vi "Prompt for Replacement.vi"(6 "Calling VI in":refnum<vi>, 8 "error in (no error)":errorcluster) -> (0 "error out":errorcluster, 2 "OK?":bool, 3 "Replace Info":T1={"Filter Column"=enum."Description", "Filter Type"=enum."Contains", "Filter Value"="", "Case Sensitive?"=FALSE, "Replace Column"=enum."Description", "Replace Value"=""})   [LabVIEW 2020, in "VI Properties Editor.lvlib"]
doc: "Displays a window to find and replace item properties."
uses:
  VI Properties Editor.lvlib
  CTLs/Filter Column.ctl
  CTLs/Filter Type.ctl
  CTLs/Replace Column.ctl
  CTLs/Replace Info.ctl
panel:
  in  "Case Sensitive?":bool caption="Case sensitive"
  in  "Replace Column Enum":T4
  in  "Replace Column":u16(ring) caption="Replacement Column" items=["Window Title", "Description", "Help Path", "Help Tag", "Custom Title?", "Help URL", "Help Type", "Control Label", "Control Caption", "Control Description", "Control Tip Strip"]
  in  "Replacement Value":string
  in  "Cancel":bool
  in  "OK":bool
  in  "Filter Type Enum":T3
  in  "Filter Type":u16(ring) items=["Contains", "Equals", "Starts with", "Ends with", "Is empty", "Does not contain", "Does not equal", "Is not empty"]
  in  "Filter Column":u16(ring) items=["Name", "Path", "Type", "Window Title", "Description", "Help Path", "Help Tag", "Custom Title?", "Reentrancy", "Inlined?", "Help URL", "Help Type", "Allow Debugging?", "Auto Error Handling?", "Run When Opened?", "Suspend When Called?", "Priority", "Preferred Exec Sytem", "Control Label", "Control Caption", "Control Description", "Control Tip Strip"]
  in  "Filter Value":string
  in  "Filter Column Enum":T2
  # "Find VIs or controls where"
  # "and change the following property to the following value:"
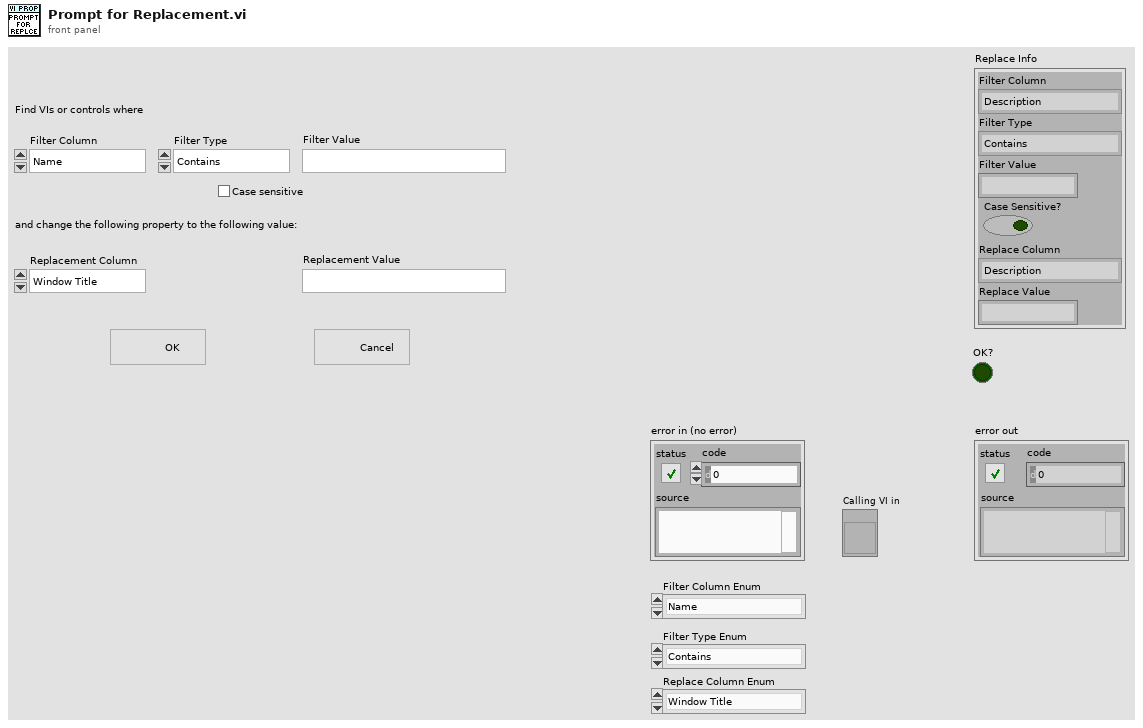
[diagram p1: front panel]
types:
  T1 = typedef "VI Properties Editor.lvlib/Replace Info.ctl" = cluster{"Filter Column":T2, "Filter Type":T3, "Filter Value":string, "Case Sensitive?":bool, "Replace Column":T4, "Replace Value":string}
  T2 = typedef "VI Properties Editor.lvlib/Filter Column.ctl" = enum16{"Name", "Path", "Type", "Window Title", "Description", "Help Path", "Help Tag", "Custom Title?", "Reentrancy", "Inlined?", "Help URL", "Help Type", "Allow Debugging?", "Auto Error Handling?", "Run When Opened?", "Suspend When Called?", "Priority", "Preferred Exec Sytem", "Control Label", "Control Caption", "Control Description", "Control Tip Strip"}
  T3 = typedef "VI Properties Editor.lvlib/Filter Type.ctl" = enum16{"Contains", "Equals", "Starts with", "Ends with", "Is empty", "Does not contain", "Does not equal", "Is not empty"}
  T4 = typedef "VI Properties Editor.lvlib/Replace Column.ctl" = enum16{"Window Title", "Description", "Help Path", "Help Tag", "Custom Title?", "Help URL", "Help Type", "Control Label", "Control Caption", "Control Description", "Control Tip Strip"}
  T5 = enum32{"Invalid", "Standard", "Closed", "Hidden", "Minimized", "Maximized"}
  T6 = enum8{"Enabled", "Disabled", "Disabled and Grayed Out"}
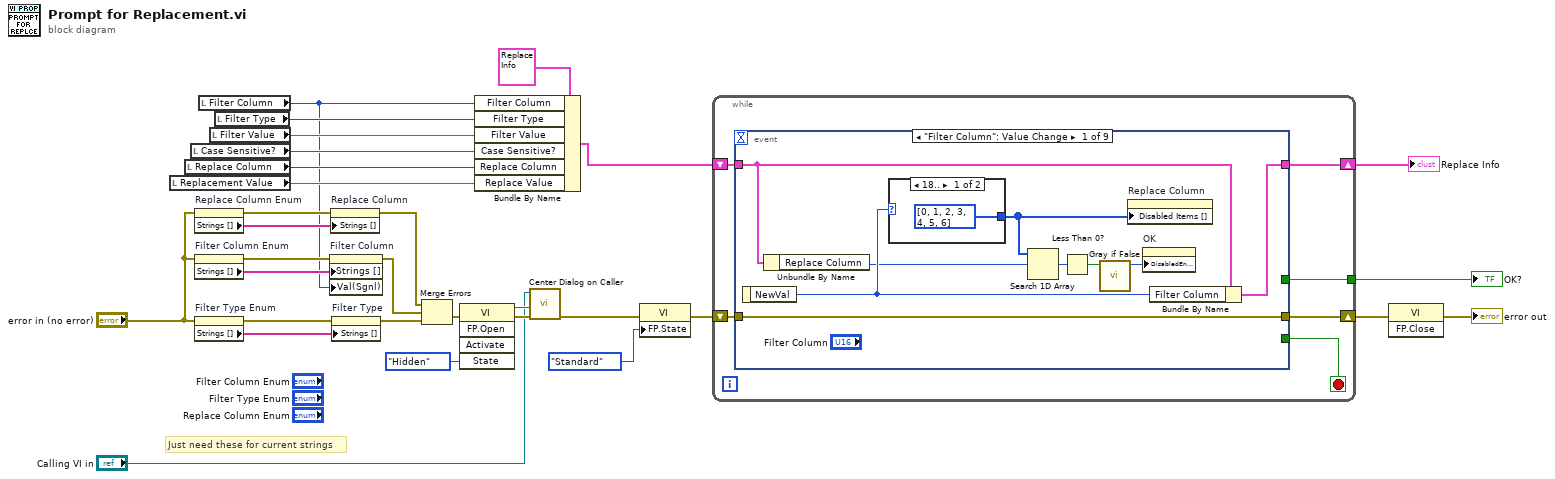
[diagram p0: block diagram]
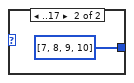
[diagram p2: hidden frame]
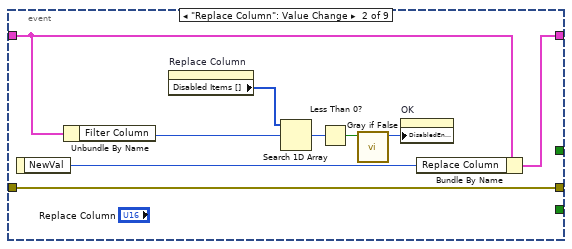
[diagram p3: hidden frame]
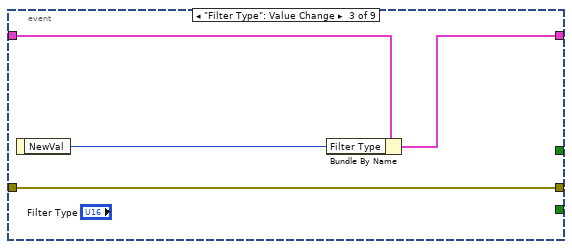
[diagram p4: hidden frame]
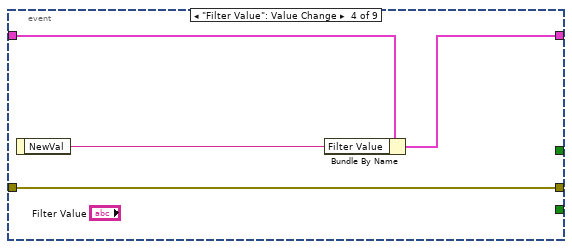
[diagram p5: hidden frame]
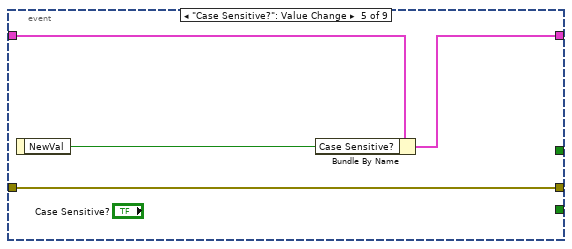
[diagram p6: hidden frame]
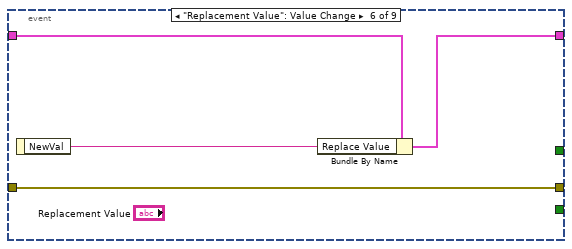
[diagram p7: hidden frame]
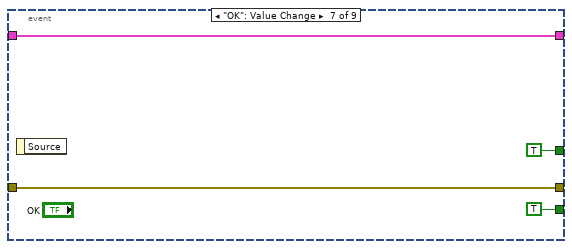
[diagram p8: hidden frame]
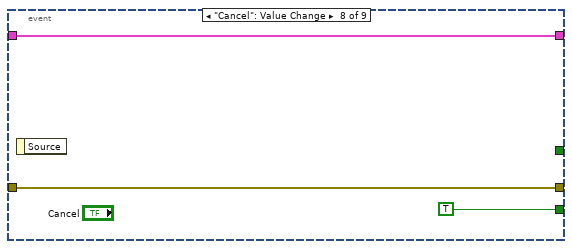
[diagram p9: hidden frame]
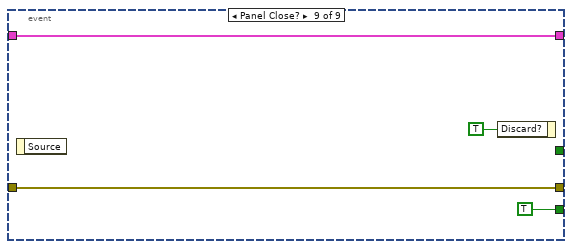
[diagram p10: hidden frame]
diagram:
  # "Just need these for current strings"
  n1 = local read "Replacement Value"() -> (w6:string)
  n2 = local read "Replace Column"() -> (w7:u16)
  n3 = local read "Case Sensitive?"() -> (w2:bool)
  n4 = property on="Replace Column Enum" class="Enum (strict)"(error in="error in (no error)") -> (error out=w18:errorcluster, "Strings []"=w5:string[])  [unwired: 1 in, 1 out]
  n5 = property on="Filter Column Enum" class="Enum (strict)"(error in="error in (no error)") -> (error out=w30:errorcluster, "Strings []"=w9:string[])  [unwired: 1 in, 1 out]
  n6 = property on="Filter Type Enum" class="Enum (strict)"(error in="error in (no error)") -> (error out=w29:errorcluster, "Strings []"=w17:string[])  [unwired: 1 in, 1 out]
  n7 = local read "Filter Column"() -> (w1:u16)
  n8 = local read "Filter Value"() -> (w15:string)
  n9 = local read "Filter Type"() -> (w14:u16)
  n10 = property on="Filter Column" class="Ring (strict)"(error in=w30, "Strings []"=w9, "Val(Sgnl)"=w1) -> (error out=w28:errorcluster)  [unwired: 1 in, 1 out]
  n11 = property on="Replace Column" class="Ring (strict)"(error in=w18, "Strings []"=w5) -> (error out=w19:errorcluster)  [unwired: 1 in, 1 out]
  n12 = property on="Filter Type" class="Ring (strict)"(error in=w29, "Strings []"=w17) -> (error out=w27:errorcluster)  [unwired: 1 in, 1 out]
  n13 = Merge Errors(w19, w28, w27) -> (w22:errorcluster)
  n14 = invoke on="Invoke Node" class="VI" method="FP.Open"(error in=w22, "State"=T5."Hidden") -> (reference out=w12:refnum<vi>, error out=w23:errorcluster)  [unwired: 3 in, 3 out]
  n15 = Bundle By Name(cluster=T1 {"Filter Column"=enum."Description", "Filter Type"=enum."Contains", "Filter Value"="", "Case Sensitive?"=FALSE, "Replace Column"=enum."Description", "Replace Value"=""} ("Replace Info"), "Filter Column"=w1, "Filter Type"=w14, "Filter Value"=w15, "Case Sensitive?"=w2, "Replace Column"=w7, "Replace Value"=w6) -> (w4:T1)
  n16 = call "Center Dialog on Caller.vi"("error in (no error)"=w23, "Dialog VI"=w12, "Calling VI in"="Calling VI in") -> ("error out"=w24:errorcluster)  [unwired: 7 in, 1 out]
  n17 = property on="Property Node" class="VI"(error in=w24, "FP.State"=T5."Standard" ("Front Panel Window:State")) -> (error out=w21:errorcluster)  [unwired: 1 in, 1 out]
  n18 = while {
    tunnel: [w31] -> w16
    shift-right: [w33] -> w3
    shift-left: w4 -> [w34]
    shift-right: [w35] -> w26
    shift-left: w21 -> [w36]
    stop <- w32 stop-if-true
    n19 = event shown="[0] \"Filter Column\": Value Change" {
      selector: _ -> [_ _ _ _ _ _ _ _ _]
      dyn-events: _ -> [_ _ _ _ _ _ _ _ _]
      timeout: _ -> [_ _ _ _ _ _ _ _ _]
      tunnel: w34 -> [w42 w53 w59 w63 w67 w71 w73 w77 w80]
      tunnel: [w44 w55 w57 w61 w65 w69 w73 w77 w80] -> w33
      tunnel: w36 -> [w45 w56 w60 w64 w68 w72 w76 w79 w83]
      tunnel: [w45 w56 w60 w64 w68 w72 w76 w79 w83] -> w35
      tunnel: [_ _ _ _ _ _ TRUE TRUE TRUE] -> w32
      tunnel: [_ _ _ _ _ _ TRUE _ _] -> w31
      event "Filter Column": Value Change {
        n20 = event-data() -> ("NewVal"=w43:u16)  [unwired: 1 in]
        n21 = Unbundle By Name(w42) -> ("Replace Column"=w40:T4)
        n22 = case shown="18.." w43 {
          tunnel: [i32[] [0, 1, 2, 3, 4, 5, 6] i32[] [7, 8, 9, 10]] -> w41
          frame 18.. {
          }
          frame ..17 {
          }
        }
        n23 = Search 1D Array(1D array=w41, element=w40) -> (index of element=w39:i32)  [unwired: 1 in]
        n24 = Less Than 0?(x=w39) -> (x < 0?=w38:bool)
        n25 = call "Gray if False.vi"("Grayed Out?"=w38) -> ("Enabled State"=w37:T6)  [unwired: 10 in]
        n26 = property on="Replace Column" class="Ring (strict)"("Disabled Items []"=w41) -> ()  [unwired: 2 in, 2 out]
        n27 = property on="OK" class="Bool"("DisabledEnum"=w37) -> ()  [unwired: 2 in, 2 out]
        n28 = Bundle By Name(cluster=w42, "Filter Column"=w43) -> (w44:T1)
      }
      event "Replace Column": Value Change {
        n29 = event-data() -> ("NewVal"=w54:u16)  [unwired: 1 in]
        n30 = Unbundle By Name(w53) -> ("Filter Column"=w52:T2)
        n31 = property on="Replace Column" class="Ring (strict)"() -> ("Disabled Items []"=w48:i32[])  [unwired: 2 in, 2 out]
        n32 = Search 1D Array(1D array=w48, element=w52) -> (index of element=w51:i32)  [unwired: 1 in]
        n33 = Less Than 0?(x=w51) -> (x < 0?=w50:bool)
        n34 = call "Gray if False.vi"("Grayed Out?"=w50) -> ("Enabled State"=w49:T6)  [unwired: 10 in]
        n35 = property on="OK" class="Bool"("DisabledEnum"=w49) -> ()  [unwired: 2 in, 2 out]
        n36 = Bundle By Name(cluster=w53, "Replace Column"=w54) -> (w55:T1)
      }
      event "Filter Type": Value Change {
        n37 = event-data() -> ("NewVal"=w58:u16)  [unwired: 1 in]
        n38 = Bundle By Name(cluster=w59, "Filter Type"=w58) -> (w57:T1)
      }
      event "Filter Value": Value Change {
        n39 = event-data() -> ("NewVal"=w62:string)  [unwired: 1 in]
        n40 = Bundle By Name(cluster=w63, "Filter Value"=w62) -> (w61:T1)
      }
      event "Case Sensitive?": Value Change {
        n41 = event-data() -> ("NewVal"=w66:bool)  [unwired: 1 in]
        n42 = Bundle By Name(cluster=w67, "Case Sensitive?"=w66) -> (w65:T1)
      }
      event "Replacement Value": Value Change {
        n43 = event-data() -> ("NewVal"=w70:string)  [unwired: 1 in]
        n44 = Bundle By Name(cluster=w71, "Replace Value"=w70) -> (w69:T1)
      }
      event "OK": Value Change {
        n45 = event-data() -> ()  [unwired: 1 in, 1 out]
      }
      event "Cancel": Value Change {
        n46 = event-data() -> ()  [unwired: 1 in, 1 out]
      }
      event Panel Close? {
        n47 = event-data() -> ()  [unwired: 1 in, 1 out]
        n48 = event-data ("Event Filter Node")("Discard?"=TRUE) -> ()  [unwired: 1 in, 1 out]
      }
    }
  }
  "OK?" <- w16
  "Replace Info" <- w3
  n49 = invoke on="Invoke Node" class="VI" method="FP.Close"(error in=w26) -> (error out=→"error out":errorcluster)  [unwired: 2 in, 2 out]
